vi "Flow Min Read Single.vi"(8 "error in":errorcluster, 9 "Channel Index":i32=1, 11 "Chiller in":refnum<class "Chiller.lvclass">) -> (0 "error out":errorcluster, 1 "Changed or First Call?":bool, 2 "Flow Min SP":dbl, 3 "Chiller out":refnum<class "Chiller.lvclass">)   [LabVIEW 2023, in "Chiller.lvclass"]
uses:
  Chiller.lvclass
  Chiller.lvclass/Chiller.ctl
  Low Level Capabilities/Flow/Flow Limit/Flow Limit.lvclass
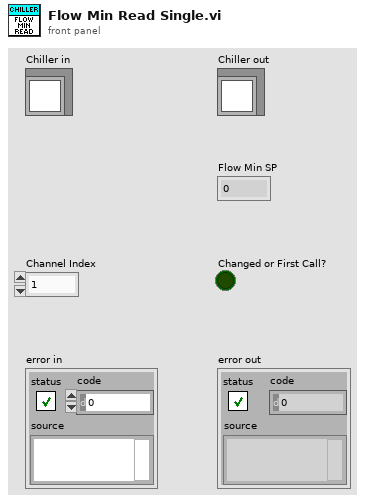
[diagram p1: front panel]
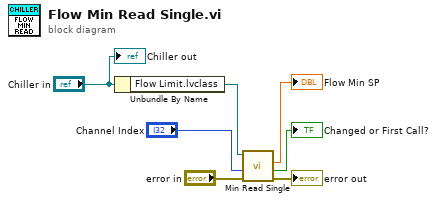
[diagram p0: block diagram]
diagram:
  n1 = Unbundle By Name("Chiller in") -> ("Flow Limit.lvclass"=w7:refnum<class "Flow Limit.lvclass">)
  n2 = call-dynamic "Min Read Single.vi"("error in"="error in", "Channel Index"="Channel Index", "Min Flow Limit in"=w7) -> ("error out"=→"error out":errorcluster, "Changed or First Call?"=→"Changed or First Call?":bool, "Flow Min SP"=→"Flow Min SP":dbl)  [unwired: 5 in, 1 out]
  "Chiller out" <- "Chiller in"
